vi "Vision Auto Gear Align.vi"(8 "Error In":errorcluster, 11 "Refnum's In":T1={"Gyro"="Gyro", "Mtr 1"="LeftMtr", "Mtr 2"="RightMtr"}) -> (0 "Error Out":errorcluster, 3 "Refnum's Out":T1={"Gyro"="Gyro", "Mtr 1"="LeftMtr", "Mtr 2"="RightMtr"})   [LabVIEW 2016]
uses:
  Robot Global Data.vi
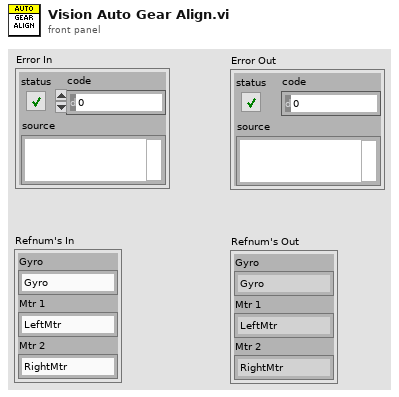
[diagram p1: front panel]
types:
  T1 = cluster{"Gyro":string, "Mtr 1":string, "Mtr 2":string}
  T2 = cluster{"Bounding Box Final":cluster{"Left":dbl, "Top":dbl, "Right":dbl, "Bottom":dbl}, "X Resolution":i32, "Y Resolution":i32}
  T3 = cluster{"Left":dbl, "Top":dbl, "Right":dbl, "Bottom":dbl}
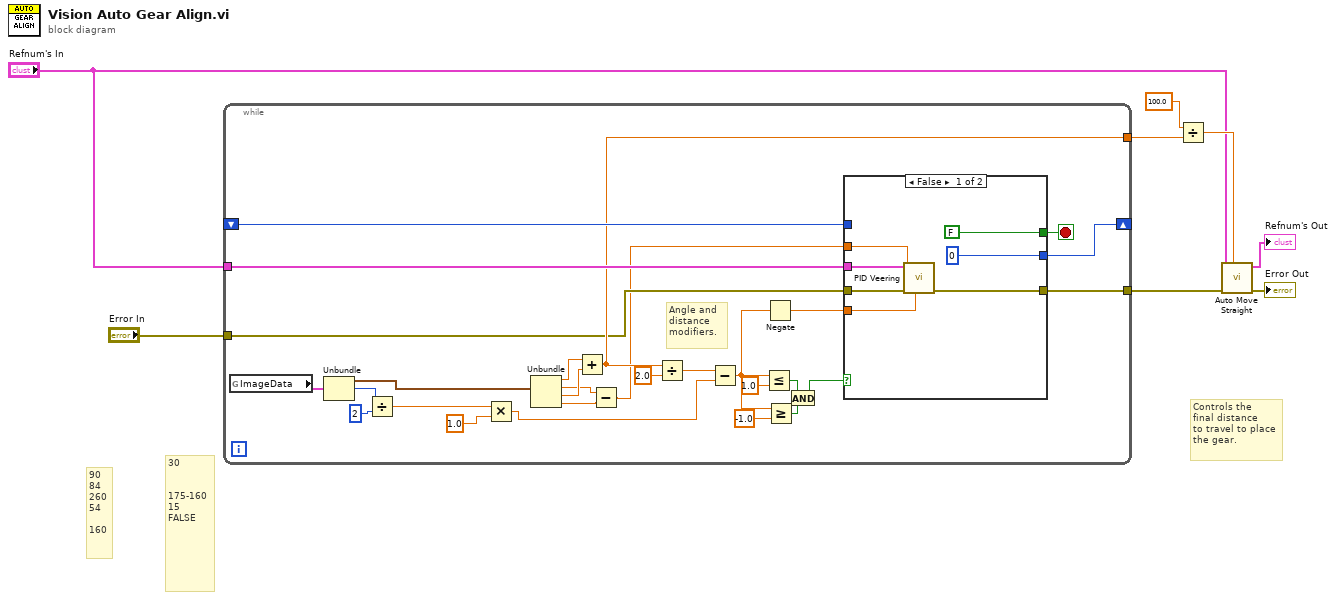
[diagram p0: block diagram]
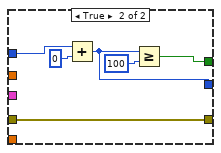
[diagram p2: hidden frame]
diagram:
  # "30\n\n\n175-160\n15\nFALSE"
  # "90\n84\n260\n54\n\n160"
  # "Controls the \nfinal distance\nto travel to place\nthe gear."
  n1 = while {
    tunnel: "Refnum's In" -> [w34]
    shift-right: [w31] -> _
    shift-left: _ -> [w30]
    tunnel: [w29] -> w2
    tunnel: "Error In" -> [w28]
    tunnel: [w27] -> w5
    stop <- w26 stop-if-true
    # "Angle and \ndistance\nmodifiers."
    n2 = global read "Robot Global Data.vi" "ImageData"() -> (w15:T2)
    n3 = Unbundle(w15) -> ("Bounding Box Final"=w14:T3, "X Resolution"=w17:i32)  [unwired: 1 out]
    n4 = Divide(x=w17, y=2) -> (x/y=w19:dbl)
    n5 = Multiply(x=w19, y=1.0) -> (x*y=w13:dbl)
    n6 = Unbundle(w14) -> ("Left"=w11:dbl, "Top"=w9:dbl, "Right"=w36:dbl, "Bottom"=w10:dbl)
    n7 = Add(x=w11, y=w36) -> (x+y=w29:dbl)
    n8 = Subtract(x=w9, y=w10) -> (x-y=w12:dbl)
    n9 = Divide(x=w29, y=2.0) -> (x/y=w33:dbl)
    n10 = Subtract(x=w33, y=w13) -> (x-y=w20:dbl)
    n11 = Less Or Equal?(x=w20, y=1.0) -> (x <= y?=w24:bool)
    n12 = Negate(x=w20) -> (-x=w21:dbl)
    n13 = Greater Or Equal?(x=w20, y=-1.0) -> (x >= y?=w23:bool)
    n14 = And(x=w24, y=w23) -> (x .and. y?=w22:bool)
    n15 = case shown="False" w22 {
      tunnel: w34 -> [w37 _]
      tunnel: w21 -> [w40 _]
      tunnel: [0 w49] -> w31
      tunnel: w30 -> [_ w48]
      tunnel: [FALSE w47] -> w26
      tunnel: w28 -> [w38 w46]
      tunnel: [w39 w46] -> w27
      tunnel: w12 -> [w41 _]
      frame False {
        n16 = call "PID Veering.vi"("Deviation"=w40, "Current Distance"=w41, "error in (no error)"=w38, "Refnum's"=w37) -> ("error out"=w39:errorcluster)  [unwired: 7 in]
      }
      frame True {
        n17 = Add(x=w48, y=0) -> (x+y=w49:i32)
        n18 = Greater Or Equal?(x=w49, y=100) -> (x >= y?=w47:bool)
      }
    }
  }
  n19 = Divide(x=100.0 ("y"), y=w2) -> (x/y=w8:dbl)
  n20 = call "Auto Move Straight.vi"("Target Distance"=w8, "Error In"=w5, "Refnum's In"="Refnum's In") -> ("Error Out"=→"Error Out":errorcluster, "Refnum's Out"=→"Refnum's Out":T1)  [unwired: 7 in]
